vi "Agilent SNA Send Cancel Pass Through.vi"(7 "Agilent SNA":T1, 8 "error in (no error)":errorcluster, 10 "Blank Frequencies (F)":bool, 11 "VISA Resource Names":T2) -> (0 "error out":errorcluster, 3 "dup VISA Resource Names":T2)   [LabVIEW 2011]
doc: "This VI for the HP8753B Network Analyzers reads the stimulus values. Except when performing log sweeps and freq list sweeps, this VI uses the start and stop values and the number of points to calcuate the stimulus values."
uses:
  TypeDefs/Agilent SNA VISA.ctl
  TypeDefs/Agilent SNA Instrument Info.ctl
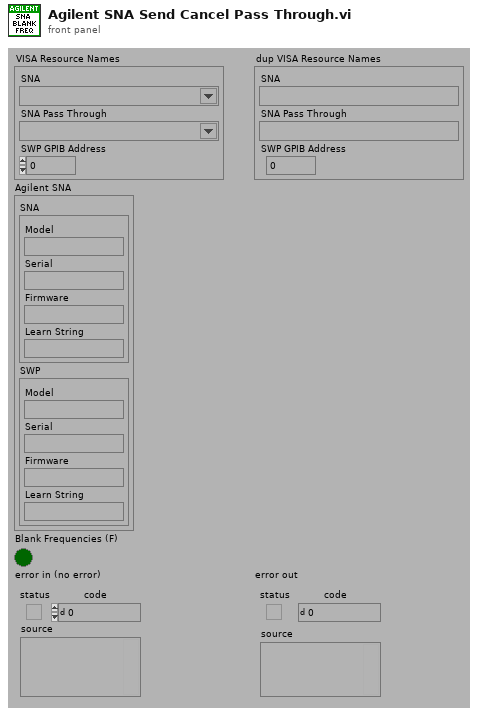
[diagram p1: front panel]
types:
  T1 = typedef "Agilent SNA Instrument Info.ctl" = cluster{"SNA":cluster{"Model":string, "Serial":string, "Firmware":string, "Learn String":string}, "SWP":cluster{"Model":string, "Serial":string, "Firmware":string, "Learn String":string}}
  T2 = typedef "Agilent SNA VISA.ctl" = cluster{"SNA":refnum<visa-resource-name>, "SNA Pass Through":refnum<visa-resource-name>, "SWP GPIB Address":i32}
  T3 = typedef "Agilent SNA Model.ctl" = enum16{"Not Supported", "8757X"}
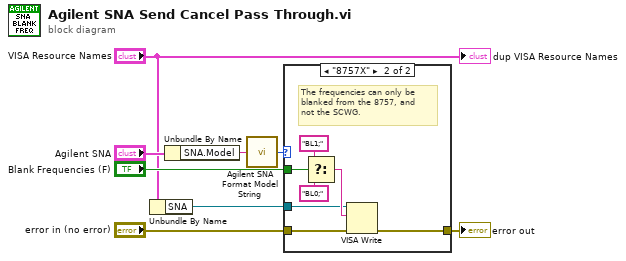
[diagram p0: block diagram]
diagram:
  n1 = Unbundle By Name("VISA Resource Names") -> ("SNA"=w1:refnum<visa-resource-name>)
  n2 = Unbundle By Name("Agilent SNA") -> ("SNA.Model"=w4:string)
  n3 = call "Agilent SNA Format Model String.vi"("Model String"=w4) -> ("Model"=w3:T3)
  n4 = case shown="\"8757X\"" w3 {
    tunnel: [w9 w12] -> w8
    tunnel: "error in (no error)" -> [w9 w13]
    tunnel: "Blank Frequencies (F)" -> [_ w10]
    tunnel: w1 -> [_ w11]
    frame "Not Supported" {
    }
    frame "8757X" {
      # "The frequencies can only be\nblanked from the 8757, and\nnot the SCWG."
      n5 = Select(t="BL1;", s=w10, f="BL0;") -> (s? t:f=w14:string)
      n6 = VISA Write(VISA resource name=w11, write buffer=w14, error in (no error)=w13) -> (error out=w12:errorcluster)  [unwired: 2 out]
    }
  }
  "error out" <- w8
  "dup VISA Resource Names" <- "VISA Resource Names"
